vi "Configure Math Calculations.vi"(8 "error in (no error)":errorcluster, 9 "Math Calculation (0: Linear)":i32(ring) items=["Linear", "Percent"], 10 "Enable Math Calculation (F: Disable)":bool, 11 "VISA resource name":refnum<visa-resource-name>) -> (0 "error out":errorcluster, 3 "VISA resource name out":refnum<visa-resource-name>)   [LabVIEW 2021, in "Keithley 2182.lvlib"]
doc: "Enables or disables math calculations and specifies which math operation to perform.\n\n1. <B>mX+b</B>: This math operation manipulates normal display readings (X) mathematically according to\nthe following calculation: <B>Y = mX+b</B>\n where:\n <B>X</B> is the normal display reading\n <B>m</B> and <B>b</B> are user-entered constants for scale factor and offset.\n <B>Y</B> is the displayed result\n\n2. <B>Percent</B>: This math function determines percent deviation from a specified reference value. The\npercent calculation is performed as follows:\n\n<B> Input - Reference\nPercent = ________________________ x 100%\n Reference\n </B>where:\n <B>Input</B> is the normal display reading\n <B>Reference</B> is the user entered constant\n <B>Percent</B> is the displayed result"
uses:
  <instrlib>/Keithley 2182/Keithley 2182.lvlib
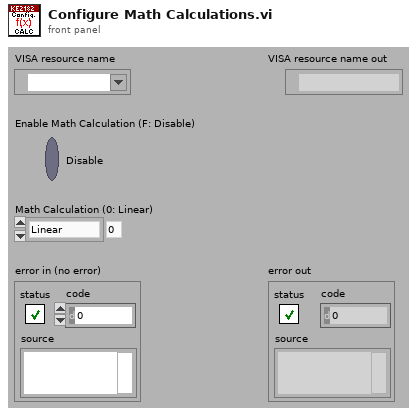
[diagram p1: front panel]
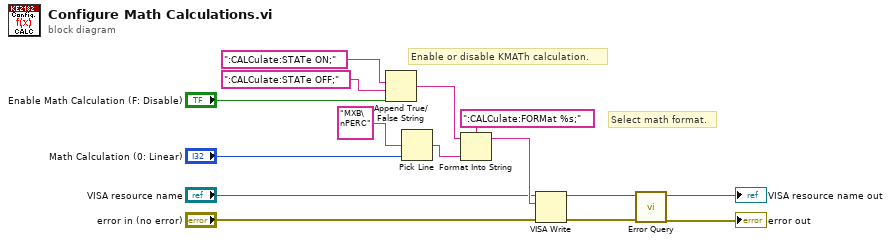
[diagram p0: block diagram]
diagram:
  # "Select math format."
  # "Enable or disable KMATh calculation."
  n1 = Append True/False String(1:"Enable Math Calculation (F: Disable)", 2:":CALCulate:STATe OFF;", 3:":CALCulate:STATe ON;") -> (0:w4:string)  [unwired: 1 in]
  n2 = Pick Line(multi-line string="MXB\nPERC", line index="Math Calculation (0: Linear)") -> (output string=w2:string)  [unwired: 1 in]
  n3 = Format Into String(format string=":CALCulate:FORMat %s;", initial string=w4, w2) -> (resulting string=w11:string)  [unwired: 1 in, 1 out]
  n4 = VISA Write(VISA resource name="VISA resource name", write buffer=w11, error in (no error)="error in (no error)") -> (VISA resource name out=w8:refnum<visa-resource-name>, error out=w7:errorcluster)  [unwired: 1 out]
  n5 = call <instrlib>:"Error Query.vi"("error in (no error)"=w7, "VISA resource name"=w8) -> ("error out"=→"error out":errorcluster, "VISA resource name out"=→"VISA resource name out":refnum<visa-resource-name>)  [unwired: 6 in, 2 out]
